vi "Count.vi"(8 "error in (no error)":errorcluster, 10 "计时":dbl=12.0 format="%0.8f", 11 "Time in":refnum<class "Time.lvclass">) -> (0 "error out":errorcluster, 1 "Time has Elapsed":bool, 2 "倒计时":dbl, 3 "Time out":refnum<class "Time.lvclass">)   [LabVIEW 2015, in "Time.lvclass"]
uses:
  Time.lvclass
  Time.lvclass/Time.ctl
panel:
  out "Elapsed Time":dbl format="%0.2f"
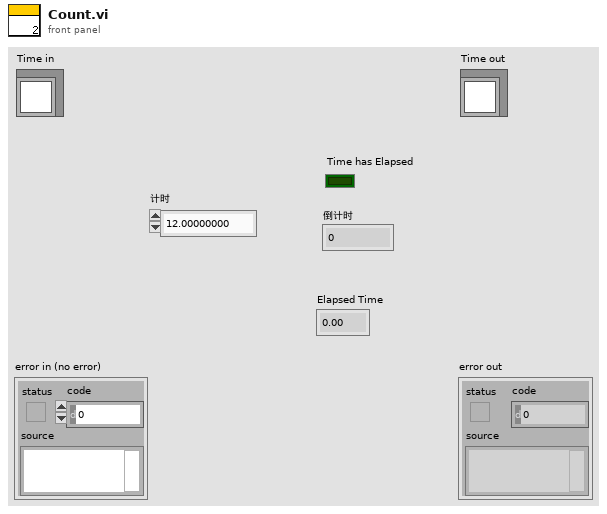
[diagram p1: front panel]
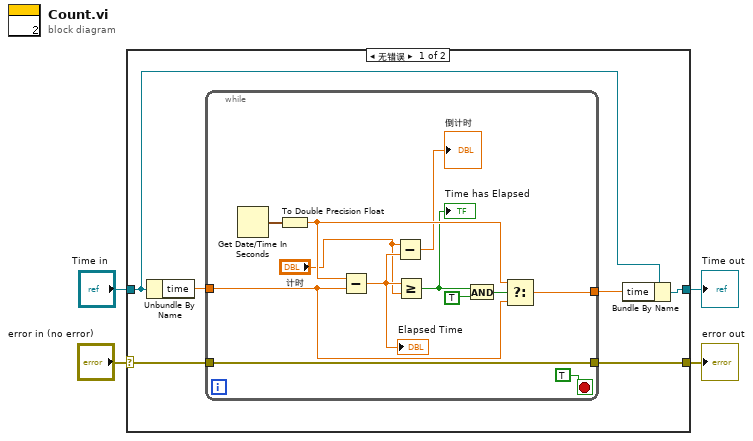
[diagram p0: block diagram]
diagram:
  n1 = case shown="无错误" "error in (no error)" {
    selector: "error in (no error)" -> [w9 w24]
    tunnel: [w8 w24] -> w3
    tunnel: [w5 w23] -> w1
    tunnel: "Time in" -> [w7 w23]
    frame No Error {
      n2 = Unbundle By Name(w7) -> ("time"=w10:dbl)
      n3 = while {
        tunnel: w10 -> [w13]
        tunnel: [w14] -> w6
        tunnel: w9 -> [w12]
        tunnel: [w12] -> w8
        stop <- TRUE stop-if-true
        n4 = Get Date/Time In Seconds() -> (seconds since 1Jan1904=w19:timestamp)
        n5 = To Double Precision Float(number=w19) -> (double precision float=w18:dbl)
        n6 = Subtract(x=w18, y=w13) -> (x-y=w17:dbl)
        "Elapsed Time" <- w17
        n7 = Subtract(x="计时", y=w17) -> (x-y=→"倒计时":dbl)
        n8 = Greater Or Equal?(x=w17, y="计时") -> (x >= y?=w16:bool)
        "Time has Elapsed" <- w16
        n9 = And(x=w16, y=TRUE ("Auto Reset")) -> (x .and. y?=w20:bool)
        n10 = Select(t=w18, s=w20, f=w13) -> (s? t:f=w14:dbl)
      }
      n11 = Bundle By Name(cluster=w7, "time"=w6) -> (w5:refnum<class "Time.lvclass">)
    }
    frame Error {
    }
  }
  "error out" <- w3
  "Time out" <- w1
